vi "SV TDMS Write Even-Angle Signal (1 Ch).vi"(0 "tdms file":refnum<k34>, 1 "write channel properties":bool=TRUE, 5 "group name in":string="Even-Angle_Signal", 7 "channel name in":string="Channel0", 9 "even-angle signal":cluster{"r0":dbl, "dr":dbl, "Y":dbl[]}={"r0"=0.0, "dr"=1.0, "Y"=[]} {"r0" format="%.2p"; "dr" format="%.2p"; "Y" format="%.2f"}, 11 "error in":errorcluster, 12 "even-angle channel info":T2={"channel name"="", "description"="", " channel info"={"sensor sensitivity"=1000.0, "engineering units"=1, "dB reference"=1.0, "custom label"="EU", "weighting filter"=0, "pregain"=0.0}} {"channel info"."pregain" format="%.2f"; "channel info"."weighting filter" items=["Linear", "A-weighting", "B-weighting", "C-weighting", "ITU-R 468-4", "Dolby", "CCITT", "C-message", "Wb", "Wc", "Wd", "We", "Wf", "Wh", "Wj", "Wk", "Wm", "AES17 20 kHz lowpass", "AES17 40 kHz lowpass", "AES17 20 kHz highpass", "AES17 40 kHz highpass"]; "channel info"."dB reference" format="%^.1e"; "channel info"."engineering units" items=["custom..."=0, "V"=1, "A"=21, "C"=30, "pC"=31, "s"=32, "-"=29, "Pa"=2, "N"=20, "g"=3, "m/s^2"=4, "m/s"=5, "m"=6, "mm/s"=12, "mm"=13, "micron/s"=14, "micron"=15, "in/s^2"=7, "in/s"=8, "in"=9, "mil/s"=10, "mil"=11, "rad/s^2"=16, "rad/s"=17, "rad"=18, "deg/s^2"=26, "deg/s"=27, "deg"=28, "RPM"=22, "cycle/s^2"=23, "Hz"=24, "cycle"=25, "strain"=19]; "channel info"."sensor sensitivity" format="%#_5f"}, 13 "even-angle position info":T1) -> (4 "tdms file out":refnum<k34>, 6 "group name out":string, 8 "channel name out":string, 15 "error out":errorcluster)   [LabVIEW 2017]
doc: "Writes data to the specified .tdms file in a format specific to the polymorphic instance. Wire data to the <B>scaled signal [EU]</B> input to determine the polymorphic instance to use or manually select the instance."
uses:
  <vilib>/addons/_NISVFA/_Shared subVIs/Controls/svc_Resampled Channel Info.ctl
  <vilib>/addons/_NISVFA/_Shared subVIs/Controls/svc_Channel Info.ctl
  <vilib>/addons/_NISVFA/_Shared subVIs/Controls/svc_Engineering Units Text Ring.ctl
  <vilib>/addons/_NISVFA/_Shared subVIs/Controls/svc_Weighting Filter Text Ring.ctl
  <vilib>/addons/_NISVFA/_Shared subVIs/Controls/svc_Position Info.ctl
  <vilib>/addons/_NISVFA/_Shared subVIs/Controls/LV Datatypes.ctl
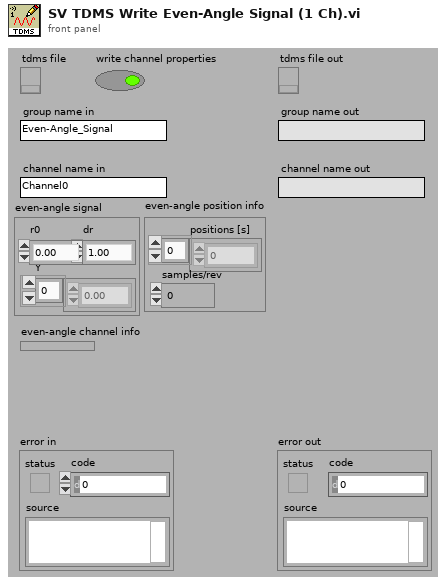
[diagram p1: front panel]
types:
  T1 = typedef "svc_Position Info.ctl" = cluster{"positions [s]":dbl[], "samples/rev":dbl}
  T2 = typedef "svc_Resampled Channel Info.ctl" = cluster{"channel name":string, "description":string, " channel info":T3}
  T3 = typedef "svc_Channel Info.ctl" = cluster{"sensor sensitivity":dbl, "engineering units":T4, "dB reference":dbl, "custom label":string, "weighting filter":T5, "pregain":dbl}
  T4 = typedef "svc_Engineering Units Text Ring.ctl" = u16
  T5 = typedef "svc_Weighting Filter Text Ring.ctl" = u16
  T6 = typedef "LV Datatypes.ctl" = i32
  T7 = typedef "NI Function Type.ctl" = u16
  T8 = typedef "NI Function SubType.ctl" = u16
  T9 = typedef "svc_X-Axis Units.ctl" = u16
  T10 = cluster{"function type":T7, "function subtype":T8, "X-domain":T9}
  T11 = typedef "svc_Unit Info.ctl" = cluster{"X-axis label":string, "X-unit string":string, "Y-axis label":string, "Y-unit string":string}
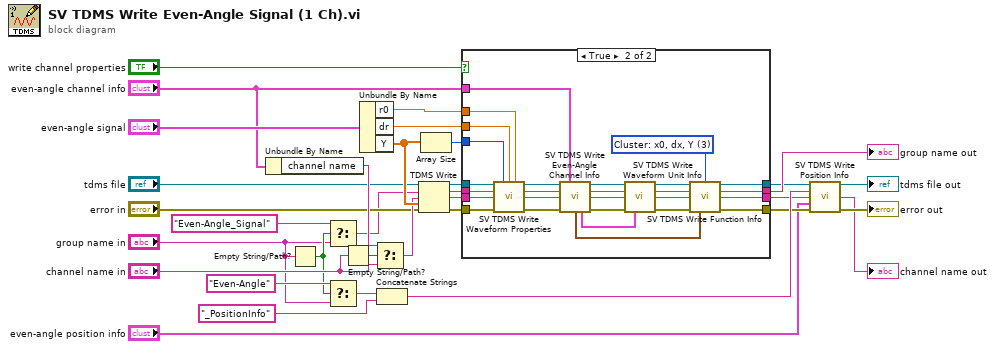
[diagram p0: block diagram]
diagram:
  n1 = Unbundle By Name("even-angle channel info") -> ("channel name"=w32:string)
  n2 = Empty String/Path?(string/path="group name in") -> (empty?=w17:bool)
  n3 = Select(t="Even-Angle_Signal", s=w17, f="group name in") -> (s? t:f=w21:string)
  n4 = Select(t="Even-Angle", s=w17, f="group name in") -> (s? t:f=w15:string)
  n5 = Empty String/Path?(string/path="channel name in") -> (empty?=w29:bool)
  n6 = Unbundle By Name("even-angle signal") -> ("r0"=w28:dbl, "dr"=w27:dbl, "Y"=w33:dbl[])
  n7 = Select(t=w32, s=w29, f="channel name in") -> (s? t:f=w31:string)
  n8 = Concatenate Strings(w15, "_PositionInfo") -> (w13:string)
  n9 = TDMS Write(0:"tdms file", 5:w21, 7:w31, 9:w33, 11:"error in") -> (4:w4:refnum<k34>, 6:w3:string, 8:w2:string, 15:w1:errorcluster)  [unwired: 1 in]
  n10 = Array Size(array=w33) -> (size(s)=w5:i32)
  n11 = case shown="True" "write channel properties" {
    tunnel: w4 -> [w37 w62]
    tunnel: w3 -> [w36 w61]
    tunnel: w2 -> [w35 w60]
    tunnel: w1 -> [w34 w59]
    tunnel: w28 -> [_ w53]
    tunnel: w27 -> [_ w54]
    tunnel: "even-angle channel info" -> [_ w64]
    tunnel: [w37 w40] -> w9
    tunnel: [w36 w39] -> w20
    tunnel: [w35 w38] -> w12
    tunnel: [w34 w41] -> w8
    tunnel: w5 -> [_ w63]
    frame False {
    }
    frame True {
      w46 = T6 3 items=["String: abc"=-2, "Boolean: True or False"=-1, "Scalar: y"=0, "Array: Y"=1, "Waveform: t0, dt, Y, variant"=2, "Cluster: x0, dx, Y"=3, "Cluster: X, Y"=4, "Waterfall"=5, "Colormap"=6] ("LabVIEW datatype")
      n12 = call <vilib>:"SV TDMS Write Waveform Properties.vi"("tdms file"=w62, "array length"=w63, "dx"=w54, "x0"=w53, "group name"=w61, "channel name"=w60, "error in (no error)"=w59) -> ("tdms file out"=w55:refnum<k34>, "group name out"=w56:string, "channel name out"=w57:string, "error out"=w58:errorcluster)  [unwired: 5 in]
      n13 = call <vilib>:"SV TDMS Write Even-Angle Channel Info.vi"("tdms file"=w55, "even-angle channel info"=w64, "group name in"=w56, "channel name in"=w57, "error in"=w58) -> ("tdms file out"=w51:refnum<k34>, "group name out"=w50:string, "channel name out"=w49:string, "function info"=w47:T10, "unit info"=w52:T11, "error out"=w48:errorcluster)  [unwired: 5 in]
      n14 = call <vilib>:"SV TDMS Write Waveform Unit Info.vi"("tdms file"=w51, "unit info"=w52, "group name"=w50, "channel name"=w49, "error in (no error)"=w48) -> ("tdms file out"=w42:refnum<k34>, "group name out"=w43:string, "channel name out"=w44:string, "error out"=w45:errorcluster)  [unwired: 7 in]
      n15 = call <vilib>:"SV TDMS Write Function Info.vi"("tdms file in"=w42, "function info"=w47, "LabVIEW datatype"=w46, "group name"=w43, "channel name"=w44, "error in (no error)"=w45) -> ("tdms file out"=w40:refnum<k34>, "group name out"=w39:string, "channel name out"=w38:string, "error out"=w41:errorcluster)  [unwired: 6 in]
    }
  }
  "group name out" <- w20
  n16 = call <vilib>:"SV TDMS Write Position Info.vi"("tdms file"=w9, "group name in"=w13, "channel name in"=w12, "speed position info"="even-angle position info", "error in (no error)"=w8) -> ("tdms file out"=→"tdms file out":refnum<k34>, "channel name out"=→"channel name out":string, "error out"=→"error out":errorcluster)  [unwired: 7 in, 1 out]
